vi "Match Longest String.vi"(3 "string array":string[](array[string]), 5 "string":string) -> (0 "index":i32, 1 "match string":string, 2 "output string":string)   [LabVIEW 2025, in "XNode Support.lvlib"]
doc: "Compares each string in <B>string array</B> with the beginning of <B>string</B>. Returns the longest of all matches."
uses:
  XNode Support.lvlib
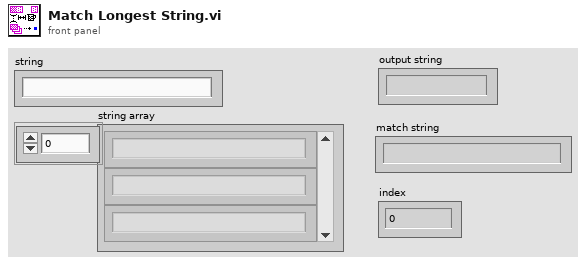
[diagram p1: front panel]
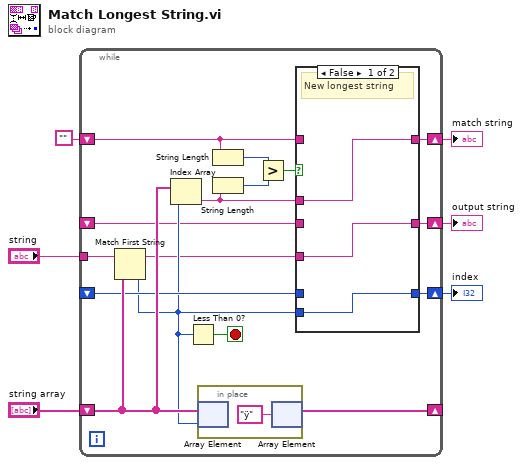
[diagram p0: block diagram]
diagram:
  n1 = while {
    tunnel: "string" -> [w22]
    shift-right: [w21] -> _
    shift-left: "string array" -> [w17]
    shift-right: [w8] -> w4
    shift-left: "" -> [w15]
    shift-right: [w7] -> w3
    shift-left: _ -> [w13]
    shift-right: [w10] -> w1
    shift-left: _ -> [w9]
    stop <- w20 stop-if-true
    n2 = Match First String(2:w17, 3:w22) -> (0:w12:i32, 1:w11:string)
    n3 = Index Array(array=w17, index=w12) -> (element=w14:string)
    n4 = Less Than 0?(x=w12) -> (x < 0?=w20:bool)
    n5 = in-place {
      n6 = in-place-array #1(w17, w12) -> ()  [unwired: 1 out]
      n7 = in-place-array #1("ÿ" ("element")) -> (w21:string[])  [unwired: 1 out]
    }
    n8 = String Length(string=w15) -> (length=w19:i32)
    n9 = String Length(string=w14) -> (length=w18:i32)
    n10 = Greater?(x=w19, y=w18) -> (0:w16:bool)
    n11 = case shown="False" w16 {
      tunnel: w15 -> [_ w28]
      tunnel: [w25 w28] -> w8
      tunnel: w14 -> [w25 _]
      tunnel: w13 -> [_ w27]
      tunnel: w12 -> [w24 _]
      tunnel: [w24 w27] -> w7
      tunnel: w11 -> [w23 _]
      tunnel: [w23 w26] -> w10
      tunnel: w9 -> [_ w26]
      frame False {
        # "New longest string"
      }
      frame True {
      }
    }
  }
  "match string" <- w4
  "index" <- w3
  "output string" <- w1
